vi "_testNewFile(AIM).vi"() -> ()   [LabVIEW 2020]
uses:
  Source/Libraries/Aim_Parameter_ni/AIM_Parameter_ni.lvlib
panel:
  in  "error in":errorcluster
  out "SerializeXML":bool
  out "error out":errorcluster
  in  "XML path":path
  in  "mode (Create)":i32(ring)=2 items=["CreateNew"=1, "Create"=2, "Open"=3, "OpenOrCreate"=4, "Truncate"=5, "Append"=6]
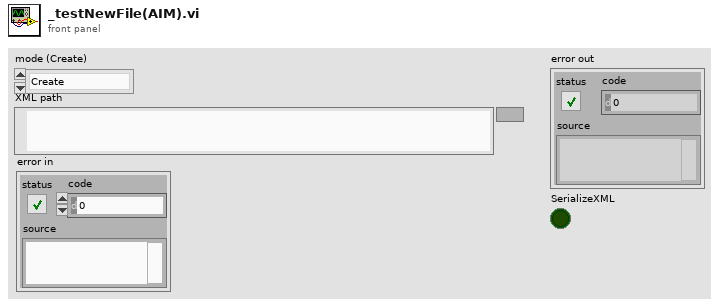
[diagram p1: front panel]
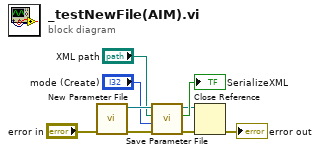
[diagram p0: block diagram]
diagram:
  n1 = call "New Parameter File.vi"("error in"="error in") -> ("error out"=w8:errorcluster, "new parameter file"=w9:refnum<k24>)  [unwired: 9 in]
  n2 = call "Save Parameter File.vi"("error in"=w8, "mode (Create)"="mode (Create)", "XML path"="XML path", "parameter file in"=w9) -> ("error out"=w5:errorcluster, "SerializeXML"=→"SerializeXML":bool, "parameter file out"=w1:refnum<k24>)  [unwired: 5 in]
  n3 = Close Reference(reference=w1, error in (no error)=w5) -> (error out=→"error out":errorcluster)
